vi "GUI_Bella_2BLMap.vi"() -> ()   [LabVIEW 2020]
uses:
  Shared/GUI_Template/GUI_master/tcp_new_data_event.ctl
  Shared/GUI_Template/GUI_master/tcp new data cluster.ctl
panel:
  in  "pos.Channel3::1":enum16{"1", "2", "3", "4", "5", "6"}(ring) caption="ProbeM6M7 FW"
  in  "pos.Channel4::1":enum16{"1", "2", "3", "4", "5", "6"}(ring) caption="F3M2 HASO FW"
  in  "pos.Channel2::1":enum16{"1", "2", "3", "4", "5", "6"}(ring) caption="F3M5 FW"
  in  "ProbeM6M7 Cam":bool caption="HPDCCD2"
  in  "F3M2 HASO":bool caption="HPDCCD2"
  in  "pos.Channel1::1":enum16{"1", "2", "3", "4", "5", "6"}(ring) caption="Shutter FW"
  in  "Position::2":dbl caption="2BL DM Iris" min=-50.0 max=50.0 format="%#_6p"
  in  "AnalogOutput.Channel 1::3":dbl caption="M4A Att" min=0.0 max=5.0 format="%#_6p"
  in  "pos.Channel0::4":enum16{"1", "2", "3", "4", "5", "6"}(ring) caption="Ghost FW"
  in  "pos.Channel0::1":enum16{"1", "2", "3", "4", "5", "6"}(ring) caption="M2A FW"
  in  "GUIdevice 4":string="FW-PL1-GHOST"
  in  "GUIdevice 3":string="ATT-2BL-M4A"
  in  "GUIdevice 2":string="IRIS-2BL-DM"
  in  "GUIdevice 1":string="FW-2BL-BTL"
  in  "Ghost Cam":bool caption="HPDCCD2"
  in  "F3M7 Cam":bool caption="HPDCCD2"
  in  "F3M5 Cam":bool caption="HPDCCD2"
  in  "F3M3 Cam":bool caption="HPDCCD2"
  in  "M4A Cam":bool caption="HPDCCD2"
  in  "2BL Shutter Cam":bool
  in  "M2A Cam":bool caption="HPDCCD2"
  in  "2BL DM Cam":bool caption="HPDCCD2"
  out "tcp data event":T1
  in  "stop":bool
  out "error IO 2":errorcluster
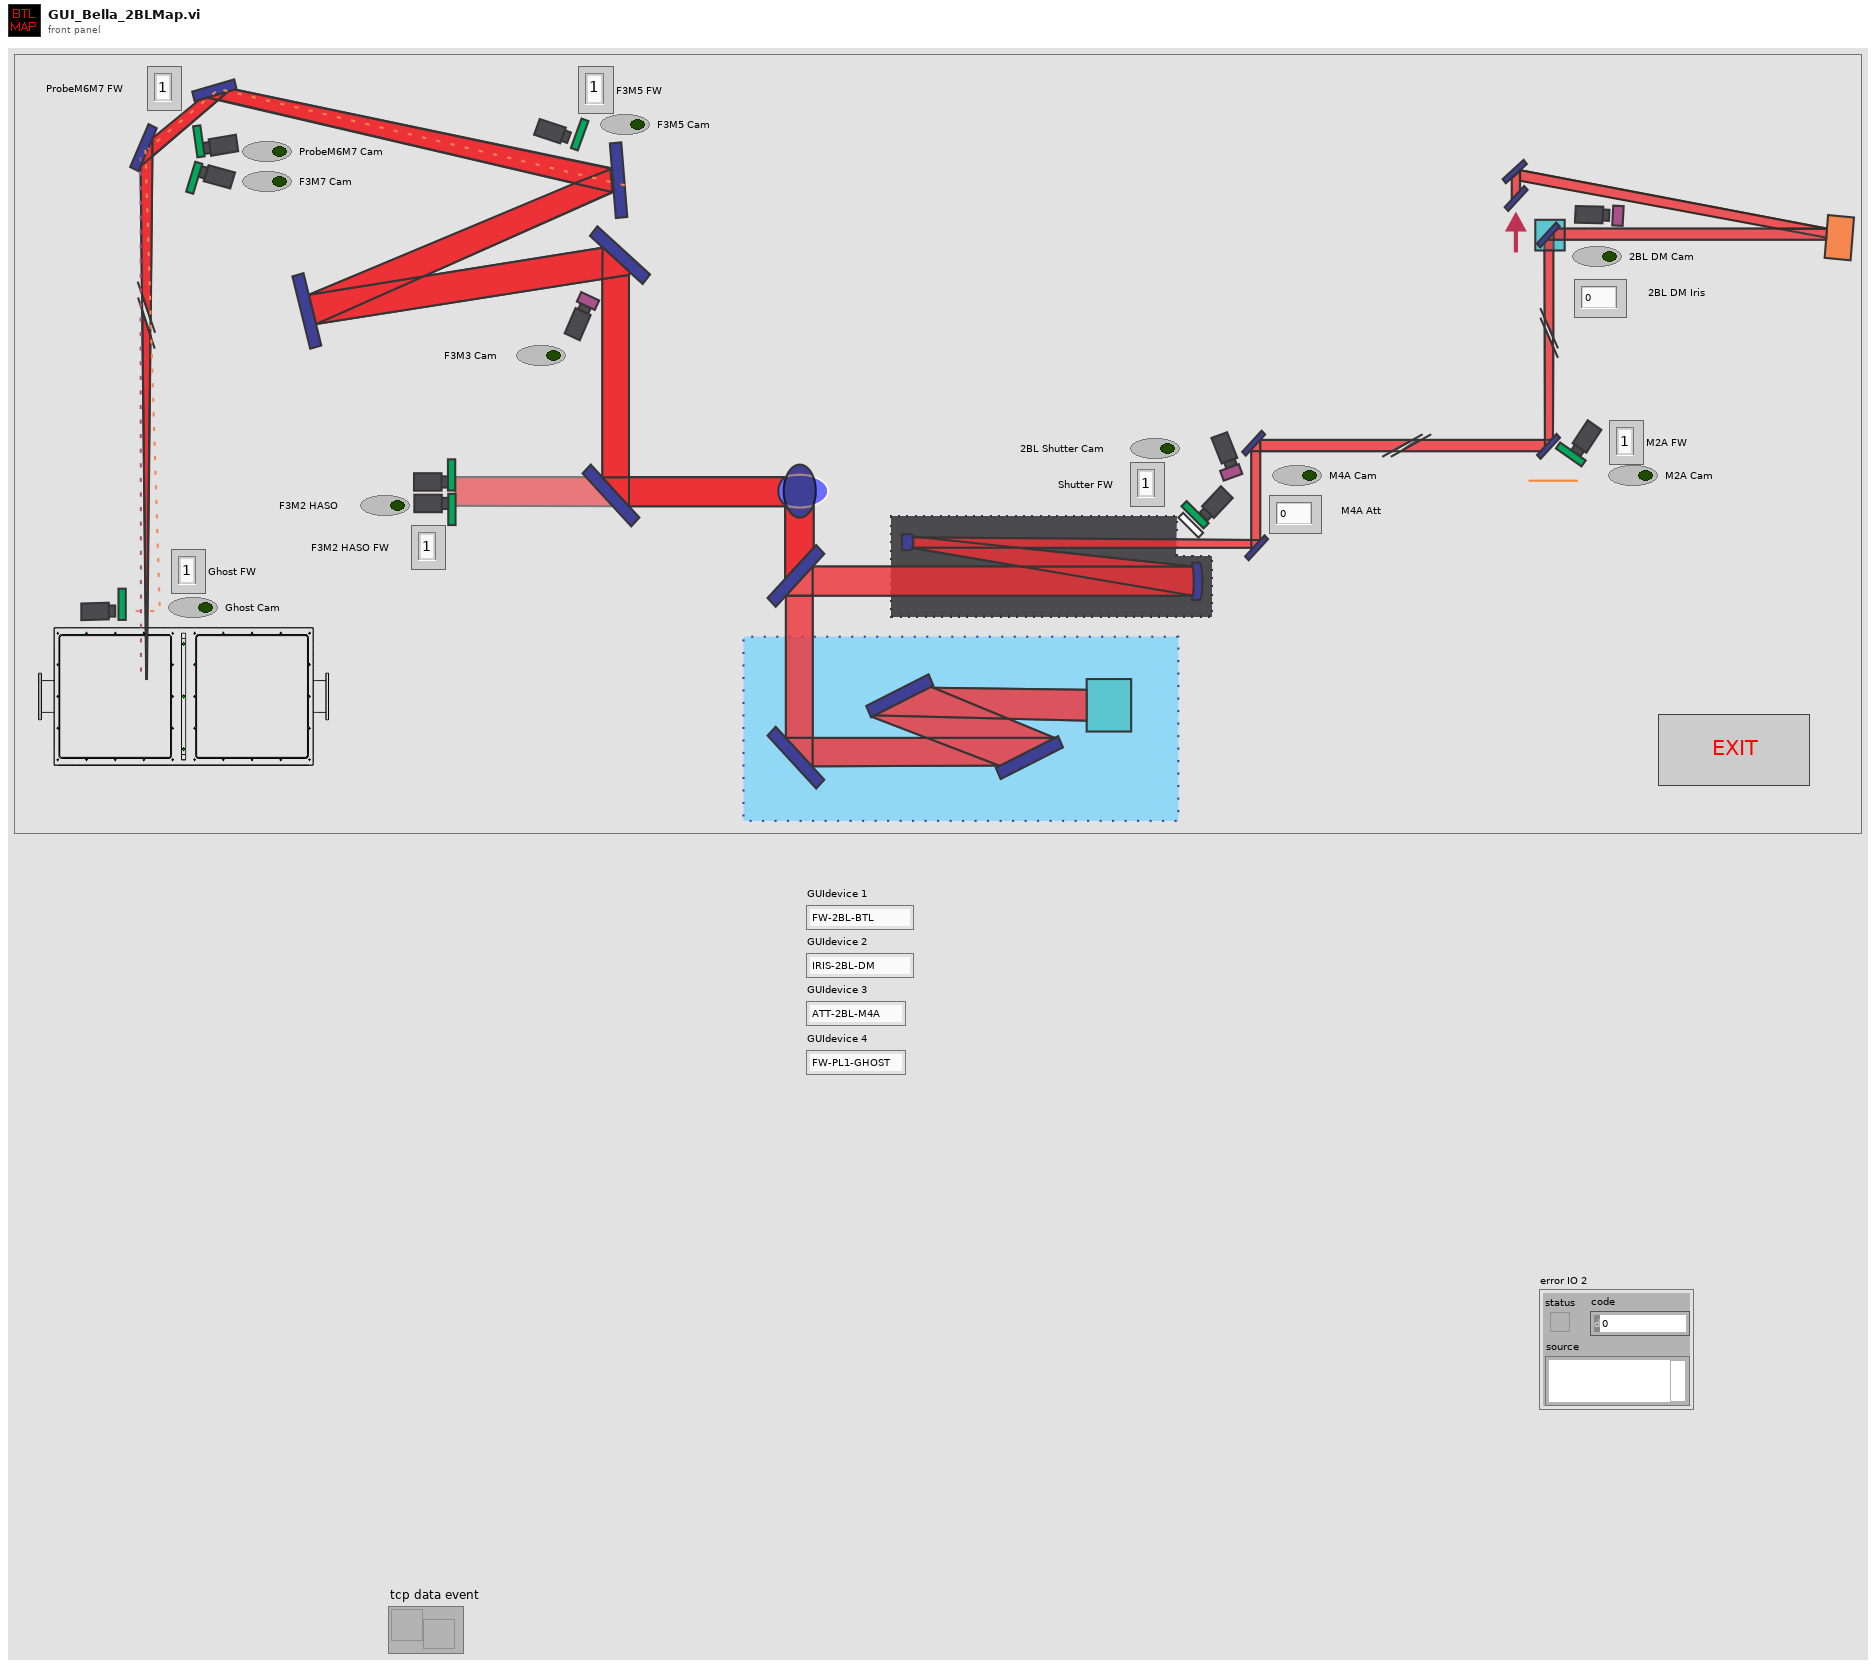
[diagram p1: front panel]
types:
  T1 = typedef "tcp_new_data_event.ctl" = refnum<user-event>
  T2 = typedef "tcp new data cluster.ctl" = cluster{"EventEnum":enum16{"new data", "connection status update"}, "Device name":string}
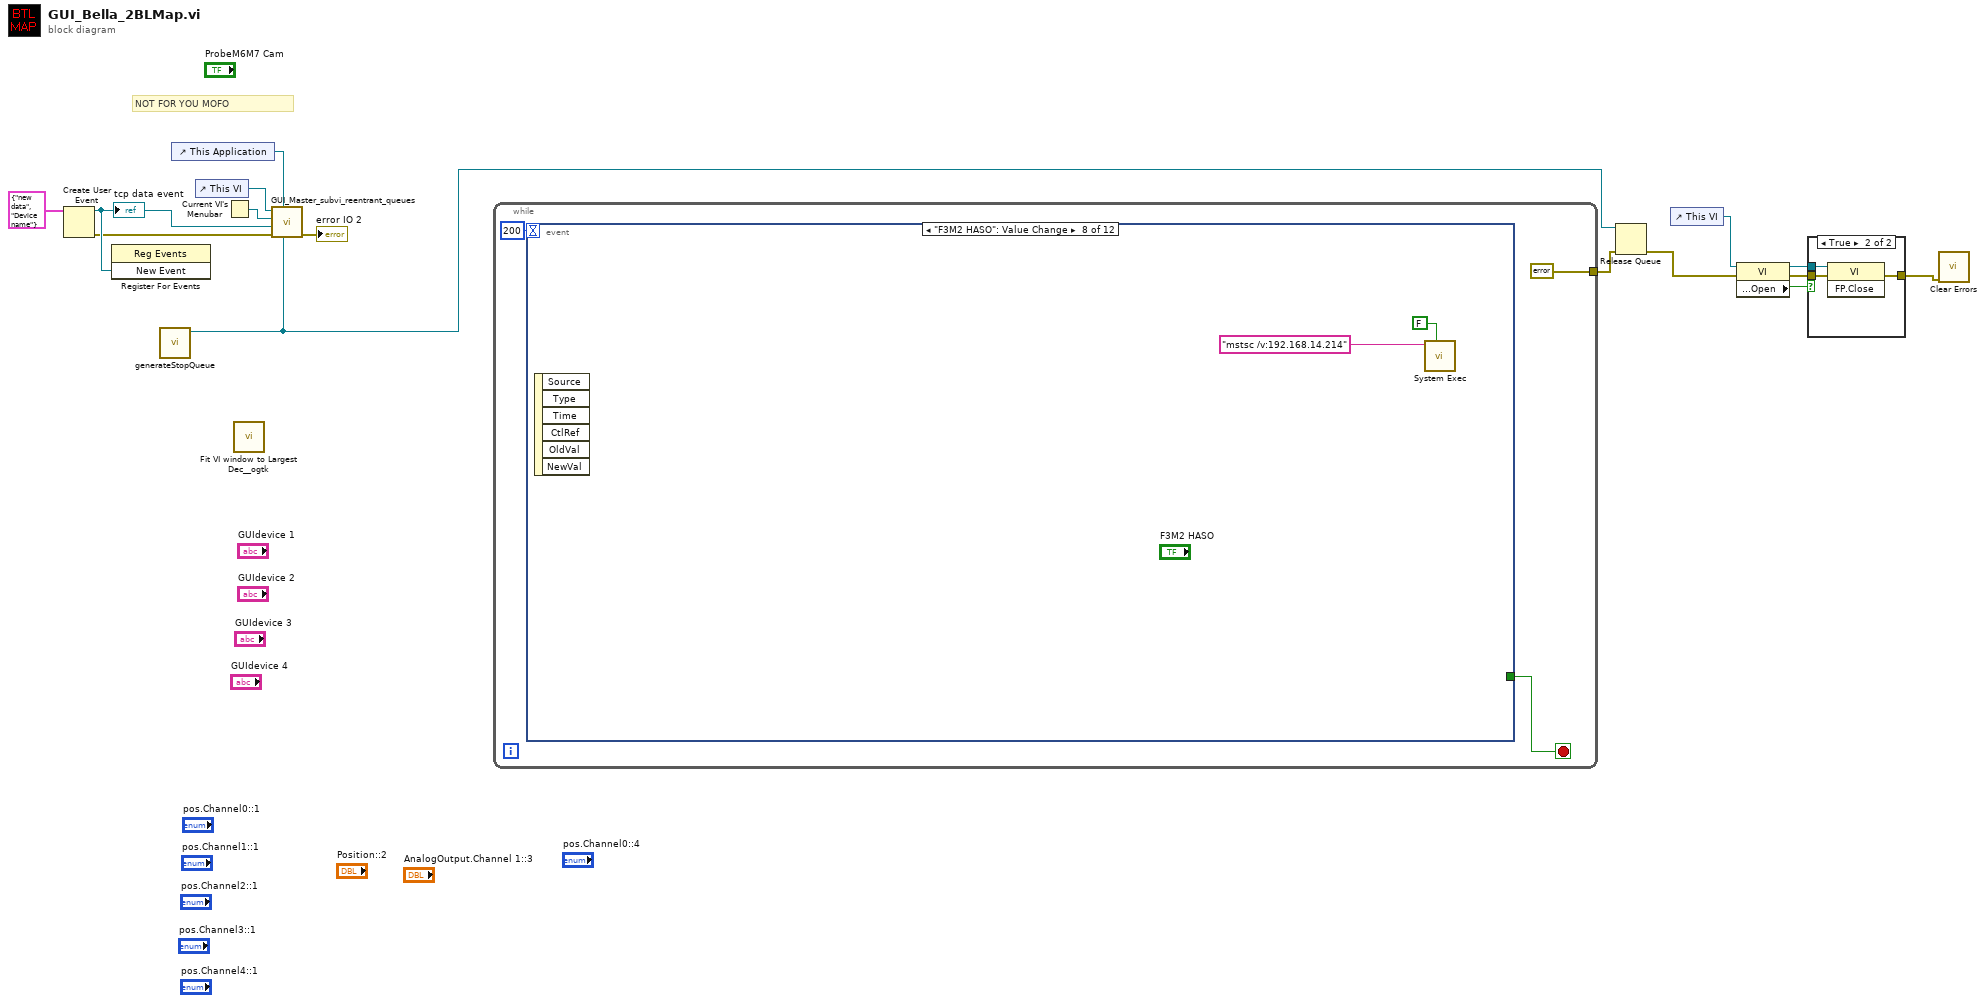
[diagram p0: block diagram]
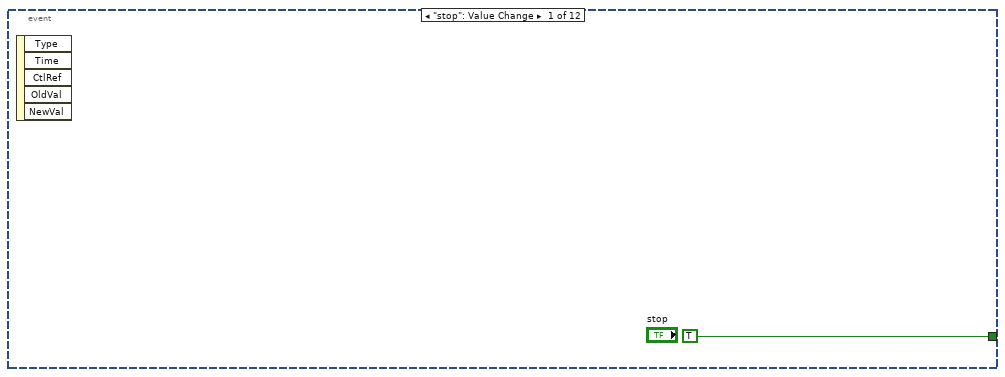
[diagram p3: hidden frame]
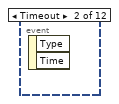
[diagram p4: hidden frame]
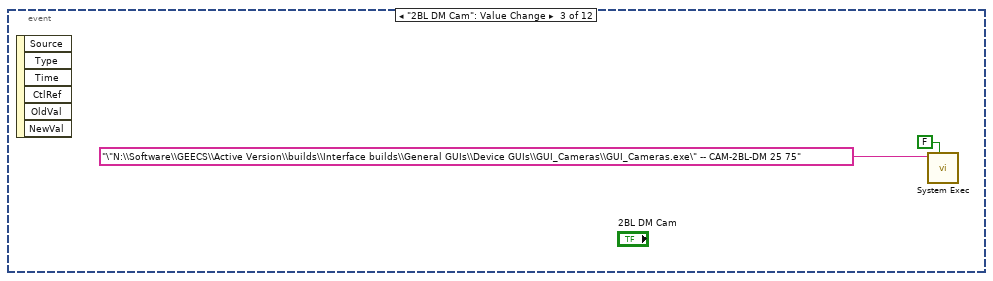
[diagram p5: hidden frame]
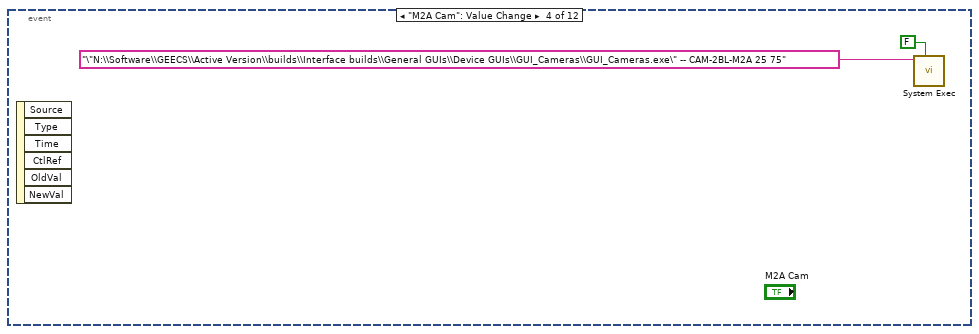
[diagram p6: hidden frame]
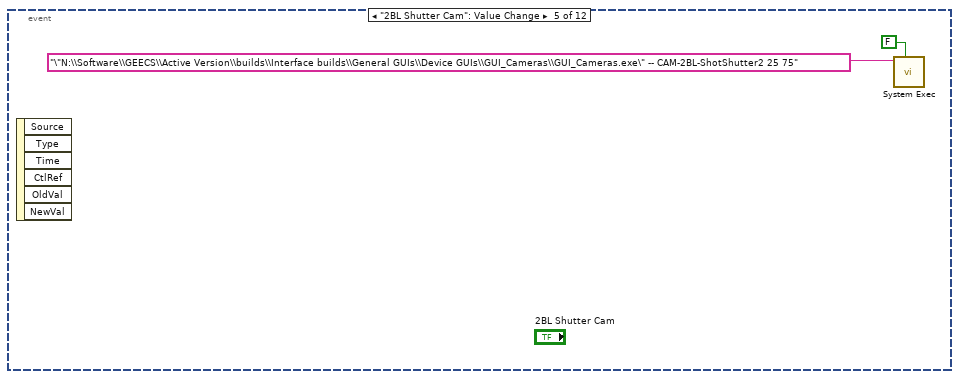
[diagram p7: hidden frame]
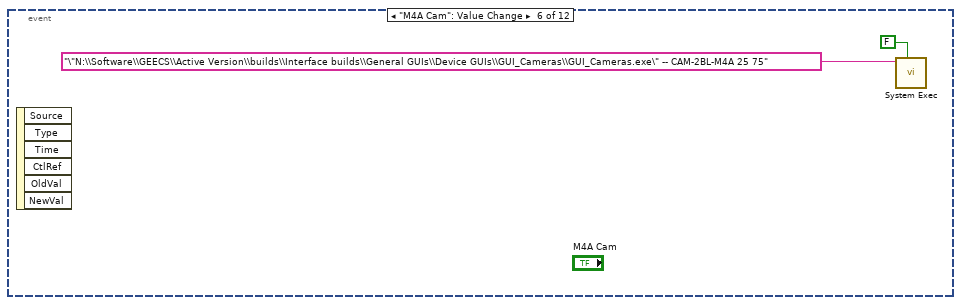
[diagram p8: hidden frame]
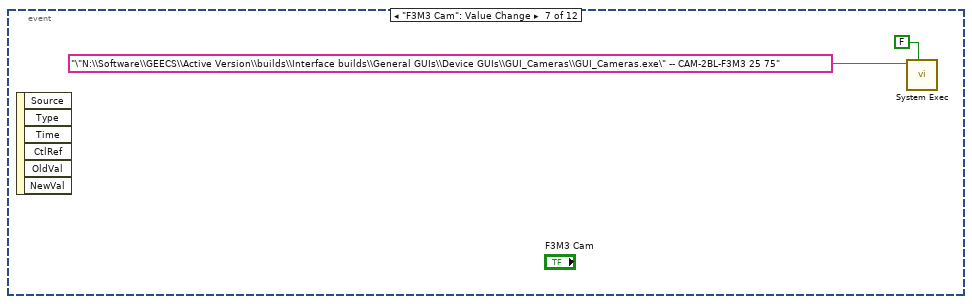
[diagram p9: hidden frame]
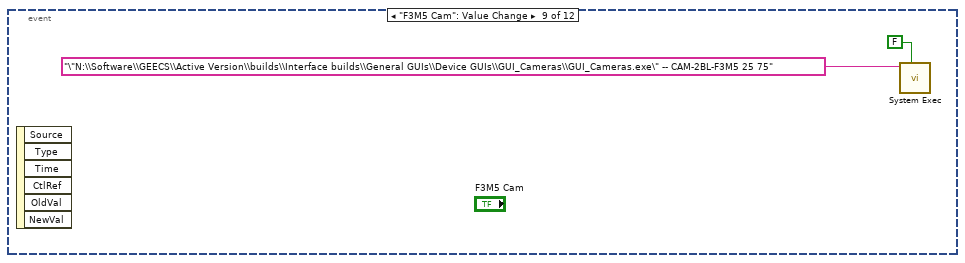
[diagram p10: hidden frame]
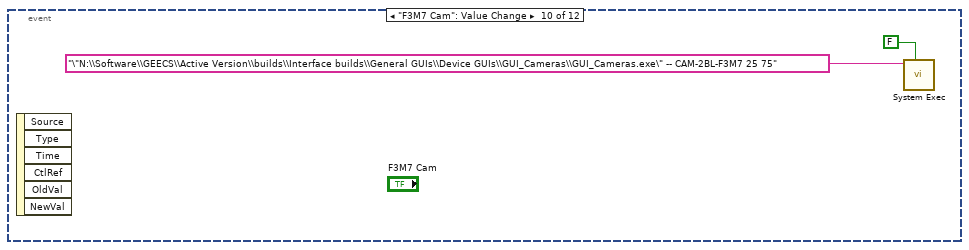
[diagram p11: hidden frame]
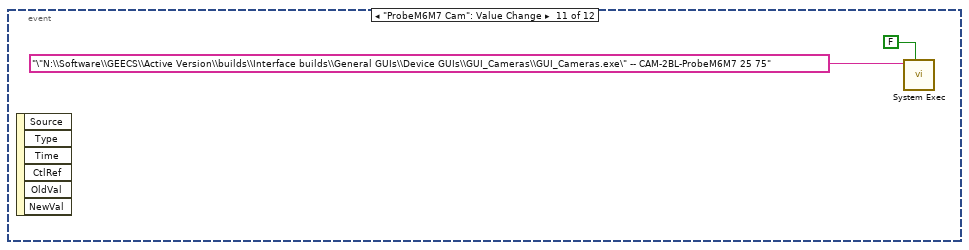
[diagram p12: hidden frame]
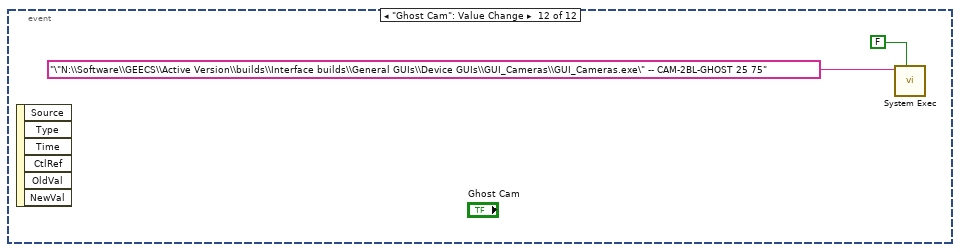
[diagram p13: hidden frame]
diagram:
  # "NOT FOR YOU MOFO"
  n1 = Create User Event(user event datatype=T2 {"EventEnum"=enum."new data", "Device name"="Device name"} ("New Event")) -> (user event=w14:refnum<user-event>, error out=w13:errorcluster)  [unwired: 1 in]
  "tcp data event" <- w14
  n2 = register-events(w14) -> ()  [unwired: 2 in, 2 out]
  n3 = call "generateStopQueue.vi"() -> ("STOP Queue out"=w8:refnum<queue>)  [unwired: 10 in, 1 out]
  n4 = control-ref of="This Application"() -> (w15:refnum<vi>)
  n5 = control-ref of="This VI"() -> (w10:refnum<vi>)
  n6 = Current VI's Menubar() -> (w11:refnum<k9>)
  n7 = call <userlib>:"Fit VI window to Largest Dec__ogtk.vi"() -> ()  [unwired: 6 in, 2 out]
  n8 = call "GUI_Master_subvi_reentrant_queues.vi"("STOP Queue in"=w8, "This Application"=w15, "error in (no error)"=w13, "tcp data event"=w14, "Caller menu reference"=w11, "Caller VI ref"=w10) -> ("error out"=→"error IO 2":errorcluster)  [unwired: 5 in]
  n9 = while {
    tunnel: [errorcluster {"status"=FALSE, "code"=0, "source"=""} ("error in (no error)")] -> w7
    stop <- w18 stop-if-true
    n10 = event shown="[7] \"F3M2 HASO\": Value Change" {
      selector: _ -> [_ _ _ _ _ _ _ _ _ _ _ _]
      dyn-events: _ -> [_ _ _ _ _ _ _ _ _ _ _ _]
      timeout: 200 -> [_ _ _ _ _ _ _ _ _ _ _ _]
      tunnel: [TRUE ("stop") _ _ _ _ _ _ _ _ _ _ _] -> w18
      event "stop": Value Change {
        n11 = event-data() -> ()  [unwired: 1 in, 5 out]
      }
      event Timeout {
        n12 = event-data() -> ()  [unwired: 1 in, 2 out]
      }
      event "2BL DM Cam": Value Change {
        n13 = event-data() -> ()  [unwired: 1 in, 6 out]
        n14 = call <vilib>:"System Exec.vi"("wait until completion? (T)"=FALSE, "command line"="\"N:\\Software\\GEECS\\Active Version\\builds\\Interface builds\\General GUIs\\Device GUIs\\GUI_Cameras\\GUI_Cameras.exe\" -- CAM-2BL-DM 25 75") -> ()  [unwired: 6 in, 4 out]
      }
      event "M2A Cam": Value Change {
        n15 = event-data() -> ()  [unwired: 1 in, 6 out]
        n16 = call <vilib>:"System Exec.vi"("wait until completion? (T)"=FALSE, "command line"="\"N:\\Software\\GEECS\\Active Version\\builds\\Interface builds\\General GUIs\\Device GUIs\\GUI_Cameras\\GUI_Cameras.exe\" -- CAM-2BL-M2A 25 75") -> ()  [unwired: 6 in, 4 out]
      }
      event "2BL Shutter Cam": Value Change {
        n17 = event-data() -> ()  [unwired: 1 in, 6 out]
        n18 = call <vilib>:"System Exec.vi"("wait until completion? (T)"=FALSE, "command line"="\"N:\\Software\\GEECS\\Active Version\\builds\\Interface builds\\General GUIs\\Device GUIs\\GUI_Cameras\\GUI_Cameras.exe\" -- CAM-2BL-ShotShutter2 25 75") -> ()  [unwired: 6 in, 4 out]
      }
      event "M4A Cam": Value Change {
        n19 = event-data() -> ()  [unwired: 1 in, 6 out]
        n20 = call <vilib>:"System Exec.vi"("wait until completion? (T)"=FALSE, "command line"="\"N:\\Software\\GEECS\\Active Version\\builds\\Interface builds\\General GUIs\\Device GUIs\\GUI_Cameras\\GUI_Cameras.exe\" -- CAM-2BL-M4A 25 75") -> ()  [unwired: 6 in, 4 out]
      }
      event "F3M3 Cam": Value Change {
        n21 = event-data() -> ()  [unwired: 1 in, 6 out]
        n22 = call <vilib>:"System Exec.vi"("wait until completion? (T)"=FALSE, "command line"="\"N:\\Software\\GEECS\\Active Version\\builds\\Interface builds\\General GUIs\\Device GUIs\\GUI_Cameras\\GUI_Cameras.exe\" -- CAM-2BL-F3M3 25 75") -> ()  [unwired: 6 in, 4 out]
      }
      event "F3M2 HASO": Value Change {
        n23 = event-data() -> ()  [unwired: 1 in, 6 out]
        n24 = call <vilib>:"System Exec.vi"("wait until completion? (T)"=FALSE, "command line"="mstsc /v:192.168.14.214") -> ()  [unwired: 6 in, 4 out]
      }
      event "F3M5 Cam": Value Change {
        n25 = event-data() -> ()  [unwired: 1 in, 6 out]
        n26 = call <vilib>:"System Exec.vi"("wait until completion? (T)"=FALSE, "command line"="\"N:\\Software\\GEECS\\Active Version\\builds\\Interface builds\\General GUIs\\Device GUIs\\GUI_Cameras\\GUI_Cameras.exe\" -- CAM-2BL-F3M5 25 75") -> ()  [unwired: 6 in, 4 out]
      }
      event "F3M7 Cam": Value Change {
        n27 = event-data() -> ()  [unwired: 1 in, 6 out]
        n28 = call <vilib>:"System Exec.vi"("wait until completion? (T)"=FALSE, "command line"="\"N:\\Software\\GEECS\\Active Version\\builds\\Interface builds\\General GUIs\\Device GUIs\\GUI_Cameras\\GUI_Cameras.exe\" -- CAM-2BL-F3M7 25 75") -> ()  [unwired: 6 in, 4 out]
      }
      event "ProbeM6M7 Cam": Value Change {
        n29 = event-data() -> ()  [unwired: 1 in, 6 out]
        n30 = call <vilib>:"System Exec.vi"("wait until completion? (T)"=FALSE, "command line"="\"N:\\Software\\GEECS\\Active Version\\builds\\Interface builds\\General GUIs\\Device GUIs\\GUI_Cameras\\GUI_Cameras.exe\" -- CAM-2BL-ProbeM6M7 25 75") -> ()  [unwired: 6 in, 4 out]
      }
      event "Ghost Cam": Value Change {
        n31 = event-data() -> ()  [unwired: 1 in, 6 out]
        n32 = call <vilib>:"System Exec.vi"("wait until completion? (T)"=FALSE, "command line"="\"N:\\Software\\GEECS\\Active Version\\builds\\Interface builds\\General GUIs\\Device GUIs\\GUI_Cameras\\GUI_Cameras.exe\" -- CAM-2BL-GHOST 25 75") -> ()  [unwired: 6 in, 4 out]
      }
    }
  }
  n33 = Release Queue(queue=w8, error in (no error)=w7) -> (error out=w2:errorcluster)  [unwired: 1 in, 2 out]
  n34 = control-ref of="This VI"() -> (w3:refnum<vi>)
  n35 = property class="VI"(reference=w3, error in=w2) -> (reference out=w5:refnum<vi>, error out=w6:errorcluster, "Front Panel.Open"=w4:bool)
  n36 = case shown="True" w4 {
    tunnel: [w40 w43] -> w1
    tunnel: w6 -> [w40 w42]
    tunnel: w5 -> [_ w41]
    frame False {
    }
    frame True {
      n37 = invoke class="VI" method="FP.Close"(reference=w41, error in=w42) -> (error out=w43:errorcluster)  [unwired: 1 in, 2 out]
    }
  }
  n38 = call <vilib>:"Clear Errors.vi"("error in (no error)"=w1) -> ()  [unwired: 5 in, 2 out]
